vi "M9347 Set Clock.vi"(8 "error in (no error)":errorcluster) -> (0 "error out":errorcluster)   [LabVIEW 2023]
panel:
  in  "VISA resource name":refnum<visa-resource-name>="TCPIP0::localhost::hislip1::INSTR"
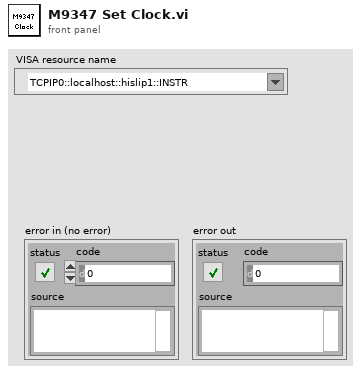
[diagram p1: front panel]
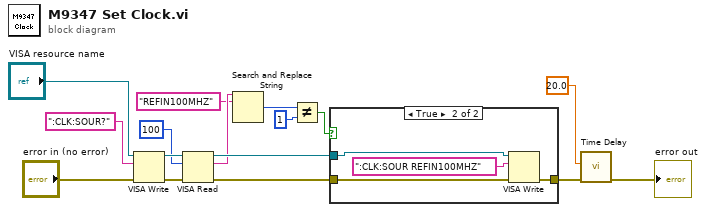
[diagram p0: block diagram]
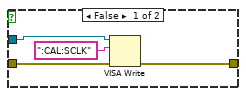
[diagram p2: hidden frame]
diagram:
  n1 = VISA Write(VISA resource name="VISA resource name", write buffer=":CLK:SOUR?", error in (no error)="error in (no error)") -> (VISA resource name out=w16:refnum<visa-resource-name>, error out=w15:errorcluster)  [unwired: 1 out]
  n2 = VISA Read(VISA resource name=w16, byte count=u32 100, error in (no error)=w15) -> (VISA resource name out=w9:refnum<visa-resource-name>, read buffer=w8:string, error out=w10:errorcluster)  [unwired: 1 out]
  n3 = Search and Replace String(input string=w8, search string="REFIN100MHZ" ("y")) -> (number of replacements=w6:i32)  [unwired: 6 in, 3 out]
  n4 = Not Equal?(x=w6, y=1) -> (x != y?=w11:bool)
  n5 = case shown="True" w11 {
    tunnel: w10 -> [w20 w24]
    tunnel: w9 -> [w18 w23]
    tunnel: [w19 w21] -> w3
    frame False {
      n6 = VISA Write(VISA resource name=w18, write buffer=":CAL:SCLK", error in (no error)=w20) -> (error out=w19:errorcluster)  [unwired: 2 out]
    }
    frame True {
      n7 = VISA Write(VISA resource name=w23, write buffer=":CLK:SOUR REFIN100MHZ" ("string"), error in (no error)=w24) -> (error out=w21:errorcluster)  [unwired: 2 out]
    }
  }
  n8 = call "Time Delay"("error in (no error)"=w3, "Delay Time (s)"=20.0) -> ("error out"=→"error out":errorcluster)  [unwired: 9 in]
